vi "PowerOff.vi"(8 "Power Supply Error IN":errorcluster, 9 "VISA resource name":refnum<visa-resource-name>, 10 "DAQ Error In":errorcluster, 11 "DAQ Channels":refnum<k21>) -> (0 "Power Supply Error":string=" INSTRUCTIONS:\r\rNormal Use:  When using subVIs that incorporate the error in/error out (or error I/O) structure, place this handler where you want to inform the user of an error, typically at the end of the I/O data path, as the last action of the program.  If the error in error? is ERROR, the handler creates a message describing the error and its source.  If the type of dialog = 1 (default), the message is displayed to the user, who can only acknowedge it.  If the type = 2, the user can acknowledge the message or abort execution; aborting a program with active I/O is not recommended.  If the type = 0, no message is displayed; this is used to process the error programmatically, and the error out cluster elements are wired to individual terminals for that reason.  \r\rOther Use:\n\r\nlocal testing.  To test the error code of a subVI or function that does not have the error I/O structure, you can wire its error code and a source string to the local error code and error source inputs.  If error in error? indicates no error and error code is not equal to 0, the local code and source are substituted for the error in values, and error? is set TRUE (ERROR).", 3 "DAQ Error":string=" INSTRUCTIONS:\r\rNormal Use:  When using subVIs that incorporate the error in/error out (or error I/O) structure, place this handler where you want to inform the user of an error, typically at the end of the I/O data path, as the last action of the program.  If the error in error? is ERROR, the handler creates a message describing the error and its source.  If the type of dialog = 1 (default), the message is displayed to the user, who can only acknowedge it.  If the type = 2, the user can acknowledge the message or abort execution; aborting a program with active I/O is not recommended.  If the type = 0, no message is displayed; this is used to process the error programmatically, and the error out cluster elements are wired to individual terminals for that reason.  \r\rOther Use:\n\r\nlocal testing.  To test the error code of a subVI or function that does not have the error I/O structure, you can wire its error code and a source string to the local error code and error source inputs.  If error in error? indicates no error and error code is not equal to 0, the local code and source are substituted for the error in values, and error? is set TRUE (ERROR).")   [LabVIEW 2018]
uses:
  <instrlib>/XP Power PLS600/XP Power PLS600.lvlib
panel:
  out "Ending Time Stamp 2":timestamp
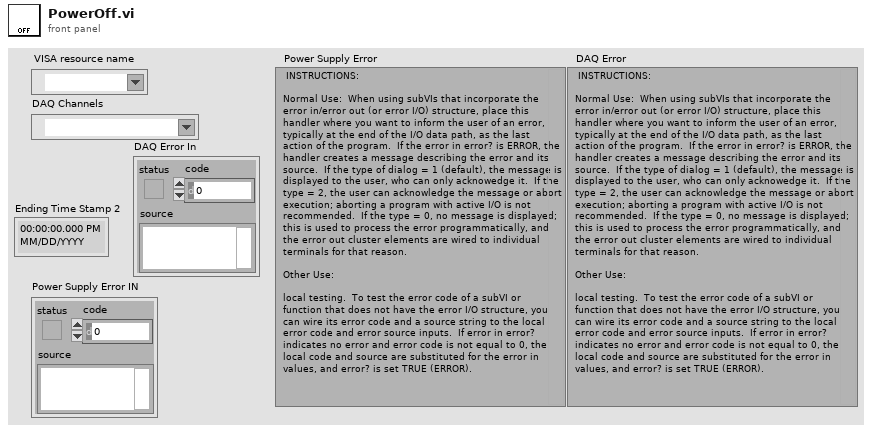
[diagram p1: front panel]
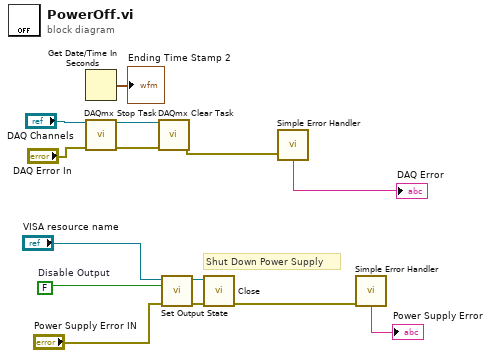
[diagram p0: block diagram]
diagram:
  w10 = FALSE  # Disable Output
  # "Shut Down Power Supply"
  n1 = Get Date/Time In Seconds() -> (seconds since 1Jan1904=→"Ending Time Stamp 2":timestamp)
  n2 = call <vilib>:"DAQmx Stop Task.vi"("task/channels in"="DAQ Channels", "error in"="DAQ Error In") -> ("task out"=w7:refnum<k21>, "error out"=w8:errorcluster)  [unwired: 12 in]
  n3 = call <vilib>:"DAQmx Clear Task.vi"("task in"=w7, "error in"=w8) -> ("error out"=w6:errorcluster)  [unwired: 13 in]
  n4 = call <instrlib>:"Set Output State.vi"("error in (no error)"="Power Supply Error IN", "Output State (F: Disable)"=w10, "VISA resource name"="VISA resource name") -> ("error out"=w11:errorcluster, "VISA resource name out"=w13:refnum<visa-resource-name>)  [unwired: 7 in]
  n5 = call <instrlib>:"Close.vi"("error in (no error)"=w11, "VISA resource name"=w13) -> ("error out"=w12:errorcluster)  [unwired: 9 in]
  n6 = call <vilib>:"Simple Error Handler.vi"("error in (no error)"=w6) -> ("message"=→"DAQ Error":string)  [unwired: 4 in, 4 out]
  n7 = call <vilib>:"Simple Error Handler.vi"("error in (no error)"=w12) -> ("message"=→"Power Supply Error":string)  [unwired: 4 in, 4 out]
